vi "BrickCollisionDetails.vi"(9 "direction in":cdb, 10 "position in":T1, 11 "class data in":refnum<class "Sprite.lvclass">) -> (3 "collisionAction out":T2)   [LabVIEW 2010, in "Labricks.lvlib" / "Brick.lvclass"]
uses:
  Brick.lvclass
  RenderBase/SceneObject_class/CollisionAction.ctl
  <vilib>/Utility/miscctls.llb/LV3DPointTypeDef.ctl
  RenderBase/Sprite_class/Sprite.lvclass
  RenderBase/SceneObject_class/SceneObject.lvclass
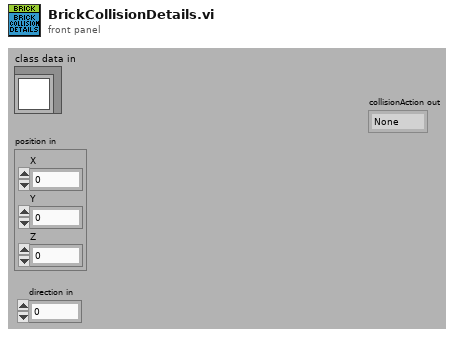
[diagram p1: front panel]
types:
  T1 = typedef "LV3DPointTypeDef.ctl" = cluster{"X":sgl, "Y":sgl, "Z":sgl}
  T2 = typedef "RenderBase.lvlib/SceneObject.lvclass/CollisionAction.ctl" = enum16{"None", "BounceX", "BounceY", "BounceXY"}
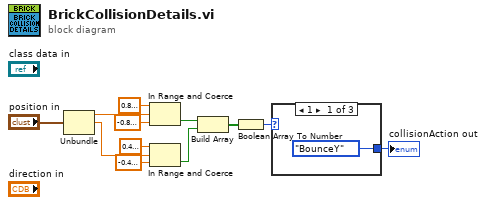
[diagram p0: block diagram]
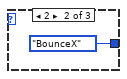
[diagram p2: hidden frame]
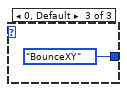
[diagram p3: hidden frame]
diagram:
  n1 = Unbundle("position in") -> ("X"=w5:sgl, "Y"=w4:sgl)  [unwired: 1 out]
  n2 = In Range and Coerce(upper limit=sgl 0.9, x=w5, lower limit=sgl -0.9) -> (In Range?=w11:bool)  [unwired: 1 out]
  n3 = In Range and Coerce(upper limit=sgl 0.4, x=w4, lower limit=sgl -0.4) -> (In Range?=w12:bool)  [unwired: 1 out]
  n4 = Build Array(w11, w12) -> (w10:bool[])
  n5 = Boolean Array To Number(Boolean array=w10) -> (number=w1:u32)
  n6 = case shown="1" w1 {
    tunnel: [CollisionAction."BounceY" ("action in") CollisionAction."BounceX" ("action in") CollisionAction."BounceXY" ("action in")] -> w2
    frame 1 {
    }
    frame 2 {
    }
    frame 0, Default {
    }
  }
  "collisionAction out" <- w2
